vi "Close.vi"(8 "error in (no error)":errorcluster caption="entrée d'erreur (pas d'erreur)", 11 "Class Relay_Board 16_Relay_CH340 en entrée":refnum<class "Class Relay_Board 16_Relay_Acer_Micro.lvclass">) -> (0 "error out":errorcluster caption="sortie d'erreur", 3 "Class Relay_Board 16_Relay_CH340 en sortie":refnum<class "Class Relay_Board 16_Relay_Acer_Micro.lvclass">)   [LabVIEW 2020, in "Library Instrument & Equipement.lvlib" / "Library Relay_Board.lvlib" / "Class Relay_Board 16_Relay_Acer_Micro.lvclass"]
uses:
  Class Relay_Board 16_Relay_Acer_Micro.lvclass
  C:/Users/ngarcin/OneDrive - Altyor/Standard TB/Class/Relay_Board/Relay_Board (Default)/Class Relay_Board (Default).lvclass
  Class Relay_Board 16_Relay_Acer_Micro.lvclass/Class Relay_Board 16_Relay_Acer_Micro.ctl
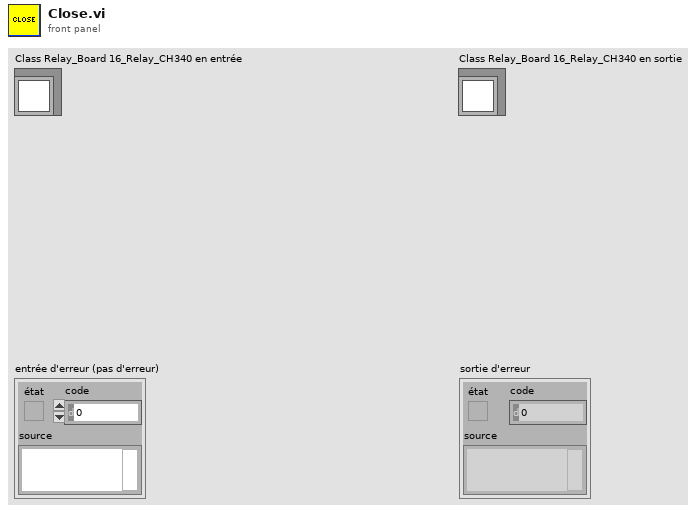
[diagram p1: front panel]
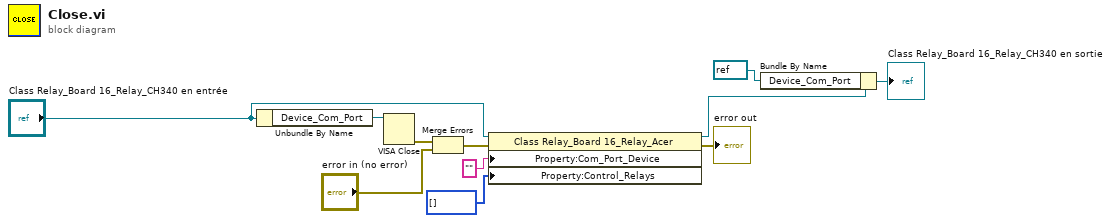
[diagram p0: block diagram]
diagram:
  n1 = Unbundle By Name("Class Relay_Board 16_Relay_CH340 en entrée") -> ("Device_Com_Port"=w7:refnum<visa-resource-name>)
  n2 = VISA Close(VISA resource name=w7) -> (error out=w10:errorcluster)  [unwired: 1 in]
  n3 = Merge Errors(w10, "error in (no error)") -> (w2:errorcluster)
  n4 = property class="Class Relay_Board 16_Relay_Acer"(reference="Class Relay_Board 16_Relay_CH340 en entrée", error in=w2, "Property:Com_Port_Device"="" ("Address_Device"), "Property:Control_Relays"=u8[] [] ("Control_Relays")) -> (reference out=w5:refnum<class "Class Relay_Board 16_Relay_Acer_Micro.lvclass">, error out=→"error out":errorcluster)
  n5 = Bundle By Name(cluster=w5, "Device_Com_Port"=refnum<visa-resource-name> refnum ("Device  @")) -> (→"Class Relay_Board 16_Relay_CH340 en sortie":refnum<class "Class Relay_Board 16_Relay_Acer_Micro.lvclass">)
